vi "Init.vi"(8 "error in (no error)":errorcluster, 10 "Channel":i16, 11 "TrialBasedExperiment in":refnum<class "TwoAfcEye.lvclass">) -> (0 "error out":errorcluster, 3 "TrialBasedExperiment out":refnum<class "TwoAfcEye.lvclass">)   [LabVIEW 2014, in "TwoAfcEye.lvclass"]
uses:
  TwoAfcEye.lvclass
  Trial Based Experiment Statechart/MatlabExperiment/MatlabExperiment.lvclass
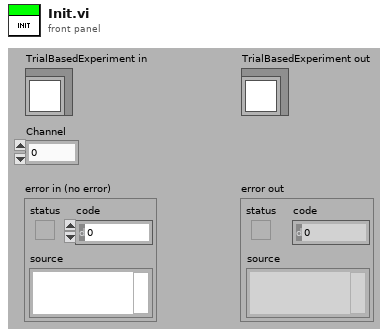
[diagram p1: front panel]
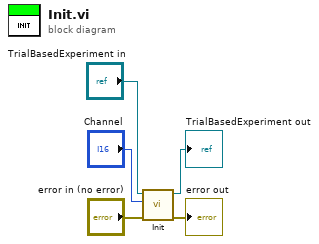
[diagram p0: block diagram]
diagram:
  n1 = call-parent "Init.vi"("error in (no error)"="error in (no error)", "Channel"="Channel", "TrialBasedExperiment in"="TrialBasedExperiment in") -> ("error out"=→"error out":errorcluster, "TrialBasedExperiment out"=→"TrialBasedExperiment out":refnum<class "TwoAfcEye.lvclass">)  [unwired: 7 in]
